vi "Curtin1_FavLists.vi"(6 "Task":enum16{"Save", "Read", "List", "Delete"}(ring), 8 "Default":string="favorites", 9 "List Name":string="favorites", 10 "description in":string, 11 "Files":T1[](array[typedef])) -> (1 "String":string, 2 "description out":string, 3 "Lists":string[](array[string]), 5 "Files Out":T1[](array[typedef]))   [LabVIEW 2022 SP3]
uses:
  Curtin1_Label.ctl
panel:
  out "error out":errorcluster
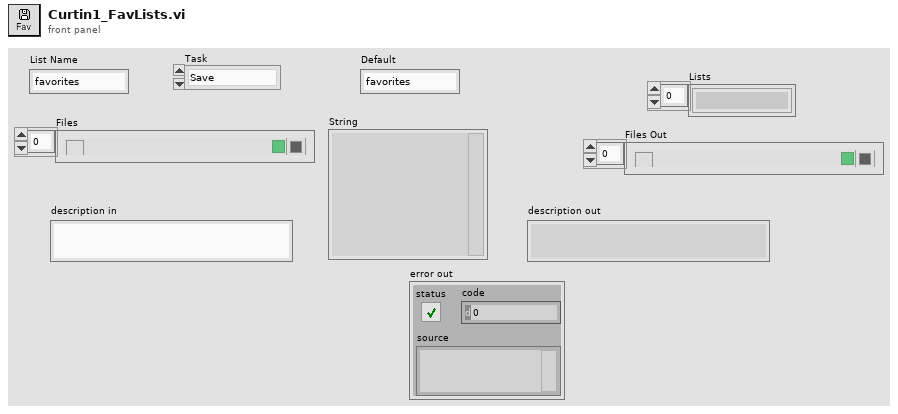
[diagram p1: front panel]
types:
  T1 = typedef "Curtin1_Label.ctl" = cluster{"Show?":bool, "Name":string, "Color":u32, "Path":path, "Show Notes":bool, "correlate":bool}
  T2 = cluster{"Show?":bool, "Name":string, "Color":u32, "Path":path, "Show Notes":bool}
  T3 = cluster{"Show?":bool, "Name":string, "Color":u32, "Path":path, "Show Notes":bool}[]
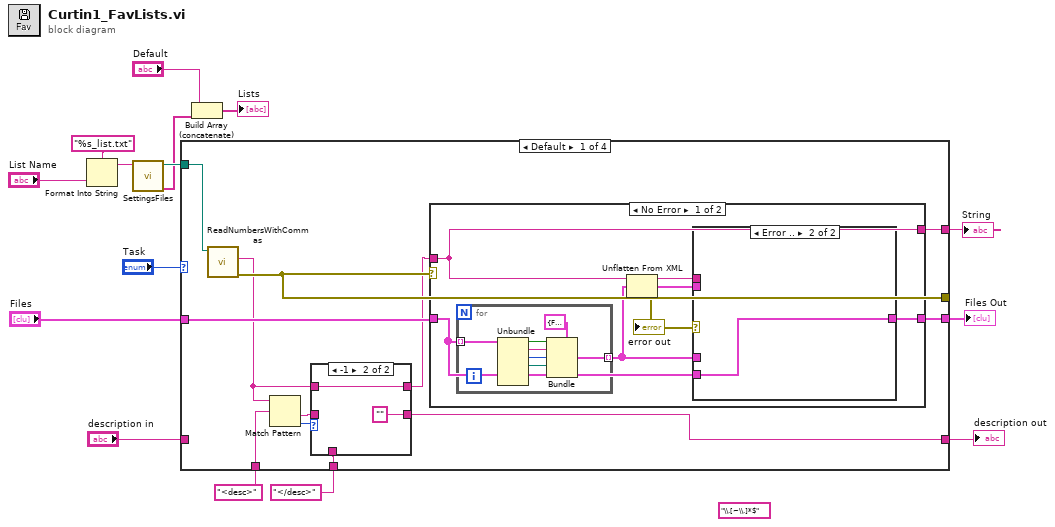
[diagram p0: block diagram]
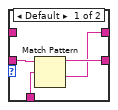
[diagram p2: hidden frame]
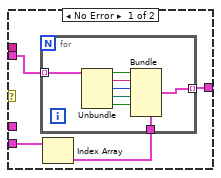
[diagram p3: hidden frame]
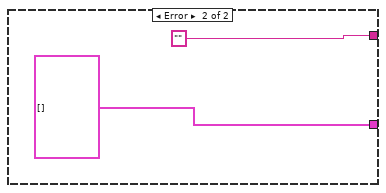
[diagram p4: hidden frame]
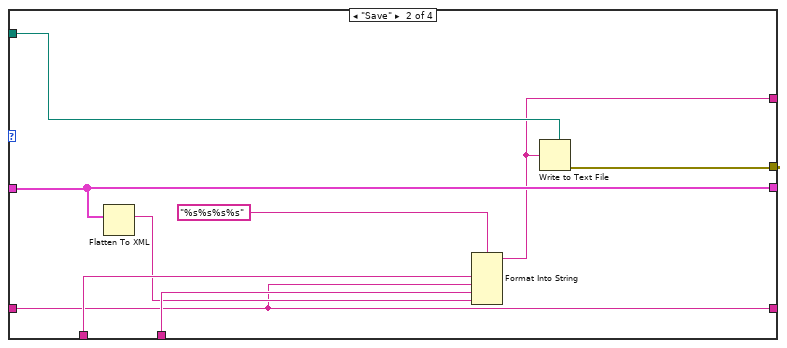
[diagram p5: hidden frame]
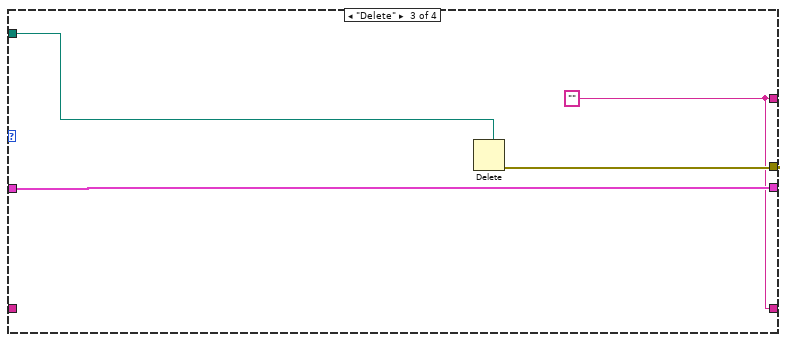
[diagram p6: hidden frame]
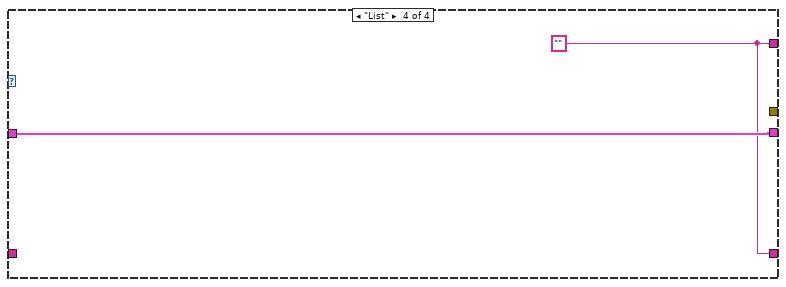
[diagram p7: hidden frame]
diagram:
  (unwired) "\\.[~\\.]*$" ("regular expression")
  n1 = Format Into String(format string="%s_list.txt" ("name or relative path"), "List Name") -> (resulting string=w4:string)  [unwired: 2 in, 1 out]
  n2 = call "SettingsFiles.vi"("settings file name"=w4) -> ("filenames"=w1:string[], "file path"=w3:path)  [unwired: 9 in]
  n3 = case shown="Default" "Task" {
    tunnel: "Files" -> [w26 w70 w74 w77]
    tunnel: [w24 w71 w75 _] -> _
    tunnel: [w27 w70 w74 w77] -> w10
    tunnel: [w25 w67 w72 w76] -> w13
    tunnel: w3 -> [w17 w69 w73 _]
    tunnel: [w18 w63 w72 w76] -> w8
    tunnel: "description in" -> [_ w63 _ _]
    tunnel: "<desc>" ("regular expression") -> [w23 w66 _ _]
    tunnel: "</desc>" ("regular expression") -> [w19 w65 _ _]
    frame Default {
      n4 = call "ReadNumbersWithCommas.vi"("file (use dialog)"=w17) -> ("error out"=w24:errorcluster, "text"=w21:string)  [unwired: 7 in, 2 out]
      n5 = Match Pattern(string=w21, regular expression=w23) -> (after substring=w20:string, offset past match=w22:i32)  [unwired: 1 in, 2 out]
      n6 = case shown="-1" w22 {
        tunnel: [w28 w33] -> w16
        tunnel: w21 -> [_ w33]
        tunnel: w20 -> [w31 _]
        tunnel: w19 -> [w30 _]
        tunnel: [w29 "" ("text")] -> w18
        frame Default {
          n7 = Match Pattern(string=w31, regular expression=w30) -> (before substring=w29:string, after substring=w28:string)  [unwired: 1 in, 2 out]
        }
        frame -1 {
        }
      }
      n8 = case shown="No Error" w24 {
        tunnel: [w35 T1[] [] ("Files")] -> w27
        tunnel: w16 -> [w38 _]
        tunnel: w26 -> [w34 _]
        tunnel: [w38 ""] -> w25
        frame No Error {
          n9 = for {
            tunnel: w34 -> [w47] mode=indexing
            tunnel: [w40] -> w36 mode=indexing
            n10 = Unbundle(w47) -> ("Show?"=w44:bool, "Name"=w45:string, "Color"=w43:u32, "Path"=w42:path, "Show Notes"=w41:bool)  [unwired: 1 out]
            n11 = Bundle(cluster=T2 {"Show?"=FALSE, "Name"="", "Color"=0, "Path"=path "", "Show Notes"=FALSE} ("Cluster"), "Show?"=w44, "Name"=w45, "Color"=w43, "Path"=w42, "Show Notes"=w41) -> (w40:T2)
          }
          n12 = Unflatten From XML(xml string=w38, type=w36) -> (value=w37:T3, error out=w39:errorcluster)  [unwired: 1 in]
          "error out" <- w39
          n13 = case shown="Error .." w39 {
            tunnel: w38 -> [_ _]
            tunnel: [w49 w60] -> w35
            tunnel: w37 -> [w51 _]
            tunnel: w36 -> [_ _]
            tunnel: w34 -> [w48 w60]
            frame No Error {
              n14 = Index Array(array=w48) -> (element=w50:T1)  [unwired: 1 in]
              n15 = for {
                tunnel: w51 -> [w59] mode=indexing
                tunnel: [w53] -> w49 mode=indexing
                tunnel: w50 -> [w52]
                n16 = Unbundle(w59) -> ("Show?"=w57:bool, "Name"=w58:string, "Color"=w56:u32, "Path"=w55:path, "Show Notes"=w54:bool)
                n17 = Bundle(cluster=w52, "Show?"=w57, "Name"=w58, "Color"=w56, "Path"=w55, "Show Notes"=w54) -> (w53:T1)  [unwired: 1 in]
              }
            }
            frame Error {
            }
          }
        }
        frame Error {
        }
      }
    }
    frame "Save" {
      n18 = Flatten To XML(6:w70) -> (2:w64:string)
      n19 = Format Into String(format string="%s%s%s%s", w66, w63, w65, w64) -> (resulting string=w67:string)  [unwired: 2 in, 1 out]
      n20 = Write to Text File(file (use dialog)=w69, text=w67) -> (error out=w71:errorcluster)  [unwired: 2 in, 2 out]
    }
    frame "Delete" {
      w72 = "" ("spreadsheet string")
      n21 = Delete(path (use dialog)=w73) -> (error out=w75:errorcluster)  [unwired: 4 in, 2 out]
    }
    frame "List" {
      w76 = "" ("spreadsheet string")
    }
  }
  "String" <- w13
  "Files Out" <- w10
  "description out" <- w8
  n22 = Build Array (concatenate)("Default", w1) -> (→"Lists":string[])
